vi "X_Y_moveSFND.vi"() -> ()   [LabVIEW 2023]
doc: "Shows how to move a motor to an absolute position."
panel:
  out "function name out":errorcluster
  out "element 2":dbl
  in  "Home 2":bool
  in  "HWSerialNum 2":i32=83829481
  in  "MG17Motor 2":refnum<k7>(container)
  out "element":dbl
  out "return value":dbl[](array[numeric])
  in  "HWSerialNum":i32=83828425
  in  "MG17Motor":refnum<k7>(container)
  in  "Stop":bool
  in  "Home":bool
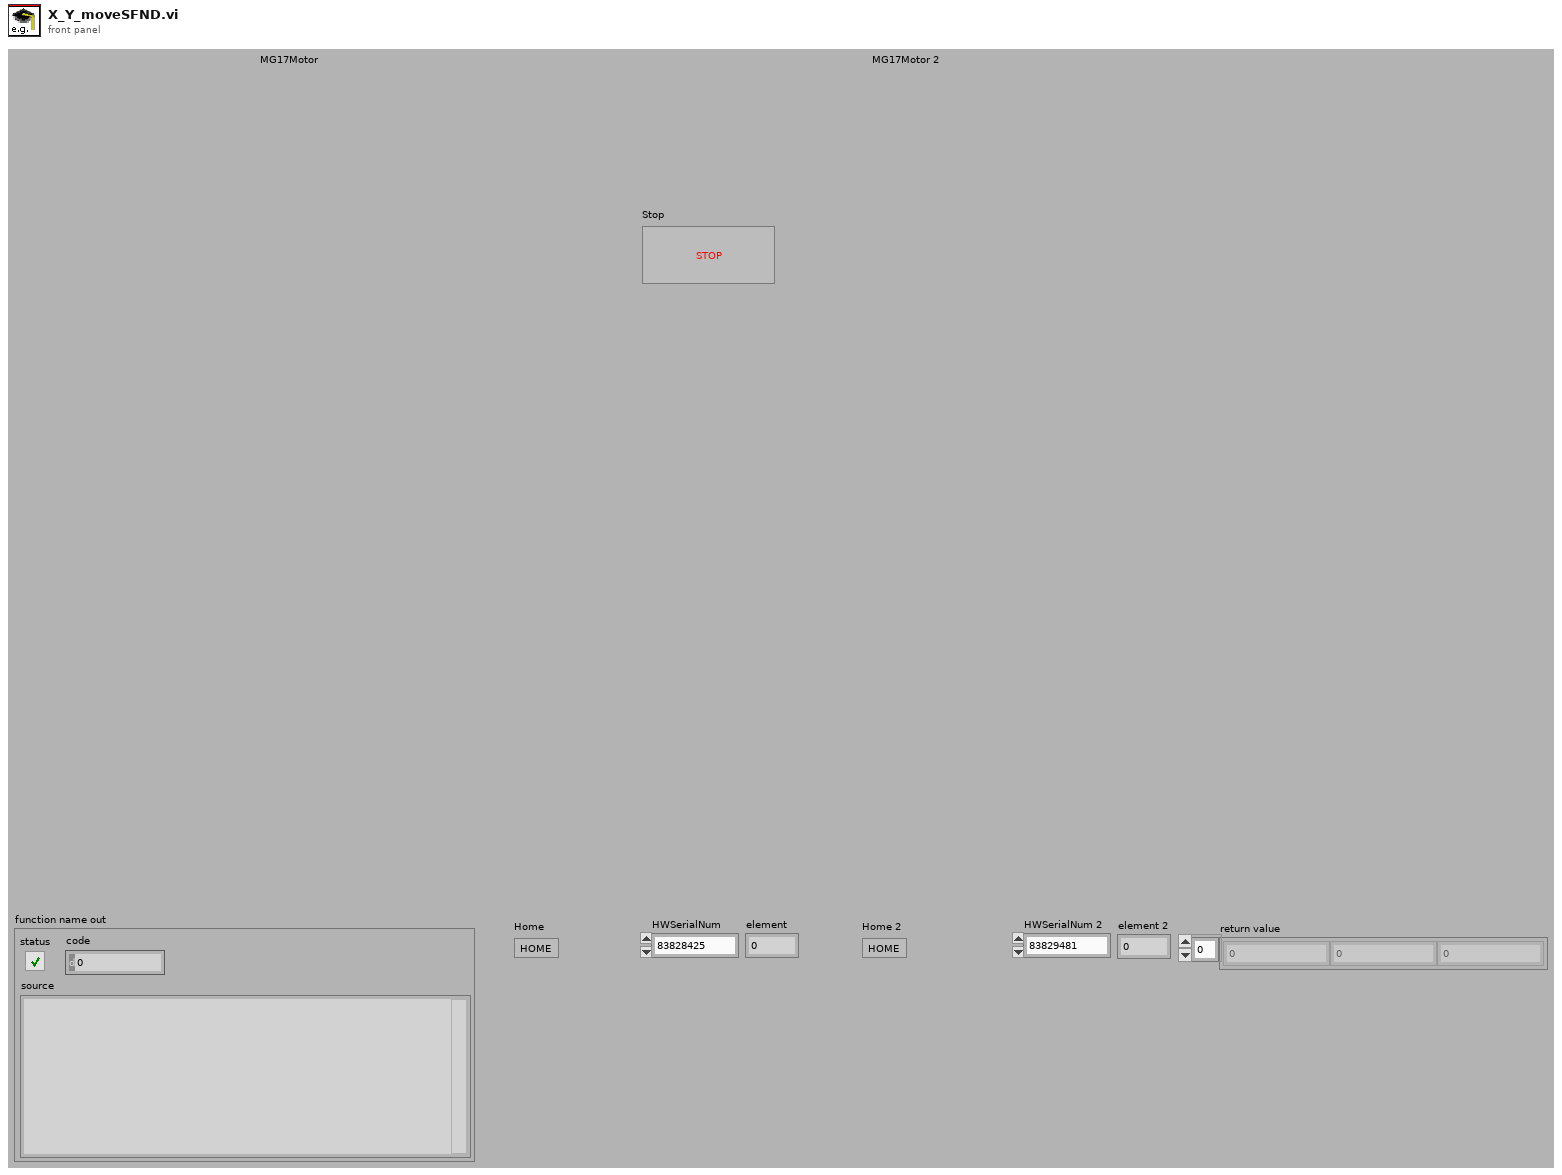
[diagram p1: front panel]
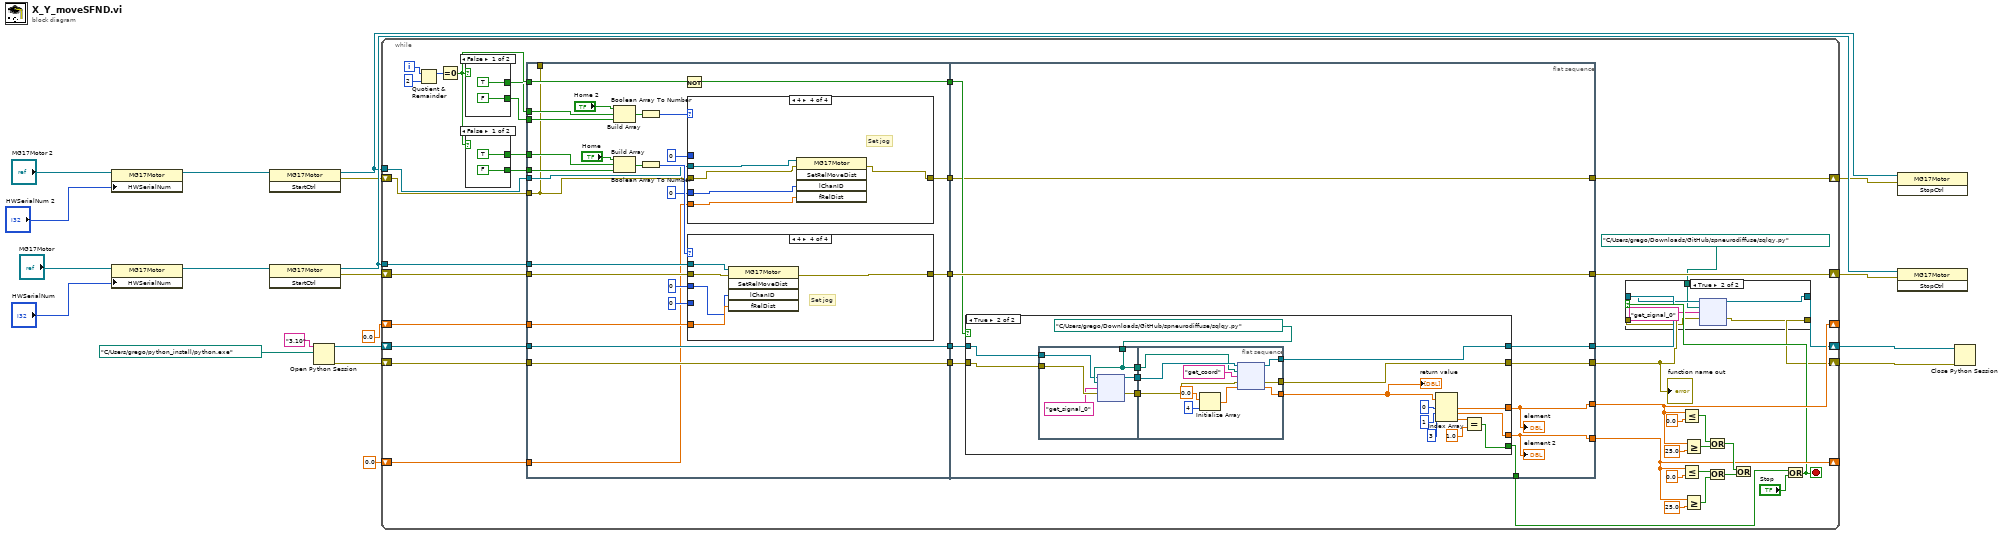
[diagram p0: block diagram]
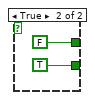
[diagram p3: hidden frame]
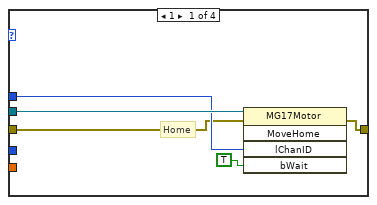
[diagram p4: hidden frame]
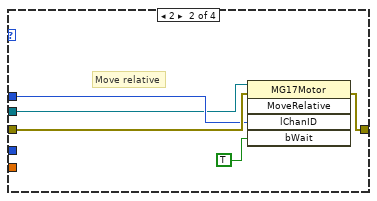
[diagram p5: hidden frame]
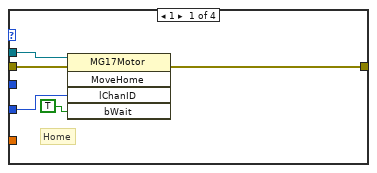
[diagram p7: hidden frame]
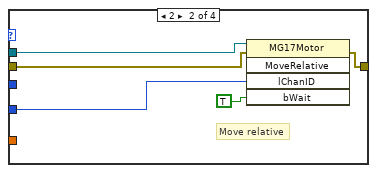
[diagram p8: hidden frame]
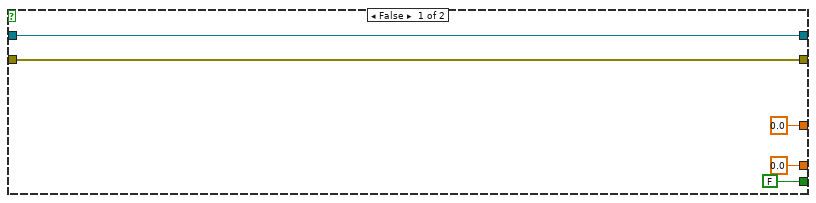
[diagram p10: hidden frame]
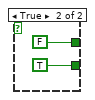
[diagram p11: hidden frame]
diagram:
  n1 = property class="MG17Motor"(reference="MG17Motor 2", "HWSerialNum"="HWSerialNum 2") -> (reference out=w8:refnum<k7>)  [unwired: 1 in, 1 out]
  n2 = property class="MG17Motor"(reference="MG17Motor", "HWSerialNum"="HWSerialNum") -> (reference out=w17:refnum<k7>)  [unwired: 1 in, 1 out]
  n3 = invoke class="MG17Motor" method="StartCtrl"(reference=w8) -> (reference out=w4:refnum<k7>, error out=w3:errorcluster)  [unwired: 2 in, 1 out]
  n4 = invoke class="MG17Motor" method="StartCtrl"(reference=w17) -> (reference out=w20:refnum<k7>, error out=w19:errorcluster)  [unwired: 2 in, 1 out]
  n5 = Open Python Session(python version="3.10" ("Python version"), python path=path "C:/Users/grego/python_install/python.exe" ("Python path")) -> (session out=w12:refnum<k35>, error out=w11:errorcluster)  [unwired: 1 in]
  n6 = while {
    shift-left: w19 -> [w61]
    shift-right: [w62] -> w18
    tunnel: w20 -> [w63]
    shift-right: [w47] -> _
    shift-left: 0.0 ("p") -> [w55]
    shift-right: [w24] -> w10
    shift-left: w12 -> [w51]
    shift-right: [w22] -> w9
    shift-left: w11 -> [w49]
    tunnel: w4 -> [w41]
    shift-right: [w32] -> _
    shift-left: 0.0 -> [w38]
    shift-right: [w31] -> w5
    shift-left: w3 -> [w30]
    i -> [w59]
    stop <- w26 stop-if-true
    n7 = Quotient & Remainder(x=w59, y=2) -> (x-y*floor(x/y)=w60:i32)  [unwired: 1 out]
    n8 = Equal To 0?(x=w60) -> (x = 0?=w42:bool)
    n9 = case shown="False" w42 {
      tunnel: [TRUE FALSE] -> w40
      tunnel: [FALSE TRUE] -> w39
      frame False {
      }
      frame True {
      }
    }
    n10 = case shown="False" w42 {
      tunnel: [TRUE FALSE] -> w57
      tunnel: [FALSE TRUE] -> w56
      frame False {
      }
      frame True {
      }
    }
    n11 = flat-sequence {
      tunnel: w63 -> [w100]
      tunnel: w61 -> [w97]
      tunnel: w57 -> [w80]
      tunnel: w56 -> [w79]
      tunnel: w55 -> [w89]
      tunnel: w42 -> [w93]
      tunnel: [w98] -> w54
      tunnel: [w92] -> w53
      tunnel: [w91] -> w52
      tunnel: w51 -> [w91]
      tunnel: [w90] -> w50
      tunnel: w49 -> [w90]
      tunnel: w41 -> [w88]
      tunnel: [w76] -> _
      tunnel: w40 -> [w86]
      tunnel: w39 -> [w85]
      tunnel: w38 -> [w77]
      tunnel: [w78] -> w37
      tunnel: w30 -> [w76]
      tunnel: [w143] -> w62
      tunnel: w54 -> [w143]
      tunnel: w53 -> [w140]
      tunnel: [w142] -> w25
      tunnel: [w141] -> w23
      tunnel: [w135] -> w47
      tunnel: w52 -> [w138]
      tunnel: w50 -> [w139]
      tunnel: w37 -> [w137]
      tunnel: [w134] -> w32
      tunnel: [w137] -> w31
      tunnel: [w136] -> w27
      frame #0 {
        n12 = Build Array("Home 2", w86, w85) -> (w84:bool[])
        n13 = Build Array("Home", w80, w79) -> (w95:bool[])
        n14 = Boolean Array To Number(Boolean array=w84) -> (number=w83:u32)
        n15 = Boolean Array To Number(Boolean array=w95) -> (number=w96:u32)
        n16 = Not(x=w93) -> (.not. x?=w92:bool)
        n17 = case shown="4" w83 {
          tunnel: w88 -> [w106 w107 _ w115]
          tunnel: 0 ("lChanID") -> [w105 w109 _ _]
          tunnel: w77 -> [_ _ _ w113]
          tunnel: [w104 w111 w112 w117] -> w78
          tunnel: w76 -> [w103 w110 w112 w116]
          tunnel: 0 ("lChanID") -> [_ _ _ w114]
          frame 1 {
            # "Home"
            n18 = invoke class="MG17Motor" method="MoveHome"(reference=w106, error in=w103, "lChanID"=w105, "bWait"=TRUE) -> (error out=w104:errorcluster)  [unwired: 1 in, 4 out]
          }
          frame 2 {
            # "Move relative"
            n19 = invoke class="MG17Motor" method="MoveRelative"(reference=w107, error in=w110, "lChanID"=w109, "bWait"=TRUE) -> (error out=w111:errorcluster)  [unwired: 1 in, 4 out]
          }
          frame Default {
          }
          frame 4 {
            # "Set jog"
            n20 = invoke class="MG17Motor" method="SetRelMoveDist"(reference=w115, error in=w116, "lChanID"=w114, "fRelDist"=w113) -> (error out=w117:errorcluster)  [unwired: 1 in, 4 out]
          }
        }
        n21 = case shown="4" w96 {
          tunnel: w100 -> [w122 w126 _ w129]
          tunnel: 0 ("lChanID") -> [w121 w124 _ _]
          tunnel: w89 -> [_ _ _ w132]
          tunnel: [w120 w127 w128 w133] -> w98
          tunnel: w97 -> [w119 w125 w128 w130]
          tunnel: 0 ("lChanID") -> [_ _ _ w131]
          frame 1 {
            # "Home"
            n22 = invoke class="MG17Motor" method="MoveHome"(reference=w122, error in=w119, "lChanID"=w121, "bWait"=TRUE) -> (error out=w120:errorcluster)  [unwired: 1 in, 4 out]
          }
          frame 2 {
            # "Move relative"
            n23 = invoke class="MG17Motor" method="MoveRelative"(reference=w126, error in=w125, "lChanID"=w124, "bWait"=TRUE) -> (error out=w127:errorcluster)  [unwired: 1 in, 4 out]
          }
          frame Default {
          }
          frame 4 {
            # "Set jog"
            n24 = invoke class="MG17Motor" method="SetRelMoveDist"(reference=w129, error in=w130, "lChanID"=w131, "fRelDist"=w132) -> (error out=w133:errorcluster)  [unwired: 1 in, 4 out]
          }
        }
      }
      frame #1 {
        n25 = case shown="True" w140 {
          tunnel: w138 -> [w148 w158]
          tunnel: w139 -> [w147 w159]
          tunnel: [w148 w153] -> w142
          tunnel: [w147 w155] -> w141
          tunnel: [0.0 w164] -> w135
          tunnel: [0.0 ("element") w162] -> w134
          tunnel: [FALSE w149] -> w136
          frame False {
          }
          frame True {
            n26 = flat-sequence {
              tunnel: path "C:/Users/grego/Downloads/GitHub/spneurodiffuse/sqlqy.py" ("module path") -> [w171]
              tunnel: [w171] -> w160
              tunnel: w159 -> [w170]
              tunnel: w158 -> [w169]
              tunnel: [w168] -> w157
              tunnel: [w167] -> w156
              tunnel: w160 -> [w173]
              tunnel: w157 -> [w174]
              tunnel: w156 -> [w172]
              tunnel: [w177] -> w155
              tunnel: [w176] -> w154
              tunnel: [w175] -> w153
              frame #0 {
                n27 = node(w169, w171, "get_signal_0" ("function name"), w170) -> (w168:refnum<k35>, w167:errorcluster)  [unwired: 2 in, 2 out]
              }
              frame #1 {
                n28 = Initialize Array(0.0 ("element"), 4 ("dimension size")) -> (w181:dbl[])
                n29 = node(w174, w173, "get_coord" ("function name"), w172, w181) -> (w175:refnum<k35>, w177:errorcluster, w176:dbl[])  [unwired: 2 out]
              }
            }
            n30 = Index Array(array=w154, index #1=0 ("index"), index #2=1 ("index"), index #3=3 ("index")) -> (element #1=w164:dbl, element #2=w162:dbl, element #3=w151:dbl)
            n31 = Equal?(x=w151, y=1.0) -> (x = y?=w149:bool)
            "return value" <- w154
          }
        }
        "element" <- w135
        "element 2" <- w134
      }
    }
    n32 = Less Or Equal?(x=w47, y=0.0) -> (x <= y?=w45:bool)
    n33 = Less Or Equal?(x=w32, y=0.0) -> (x <= y?=w34:bool)
    n34 = Greater Or Equal?(x=w47, y=25.0) -> (x >= y?=w44:bool)
    n35 = Greater Or Equal?(x=w32, y=25.0) -> (x >= y?=w33:bool)
    n36 = Or(x=w45, y=w44) -> (x .or. y?=w43:bool)
    n37 = Or(x=w34, y=w33) -> (x .or. y?=w29:bool)
    n38 = Or(x=w43, y=w29) -> ()  [unwired: 1 out]
    n39 = Or(x=w27, y="Stop") -> (x .or. y?=w26:bool)
    n40 = case shown="True" w26 {
      tunnel: w25 -> [w65 w71]
      tunnel: [w65 w66] -> w24
      tunnel: w23 -> [w64 w69]
      tunnel: [w64 w67] -> w22
      tunnel: path "C:/Users/grego/Downloads/GitHub/spneurodiffuse/sqlqy.py" ("module path") -> [_ w68]
      frame False {
      }
      frame True {
        n41 = node(w71, w68, "get_signal_0" ("function name"), w69) -> (w66:refnum<k35>, w67:errorcluster)  [unwired: 2 in, 2 out]
      }
    }
    "function name out" <- w23
  }
  n42 = invoke class="MG17Motor" method="StopCtrl"(reference=w4, error in=w5) -> ()  [unwired: 1 in, 3 out]
  n43 = invoke class="MG17Motor" method="StopCtrl"(reference=w20, error in=w18) -> ()  [unwired: 1 in, 3 out]
  n44 = Close Python Session(session in=w10, error in=w9) -> ()  [unwired: 1 out]
